vi "Populate gRPC Events.vi"(7 "RPC Method Parameters":T1[](array[typedef]), 8 "error in (no error)":errorcluster, 11 "Server class in":refnum<vi>) -> (0 "error out":errorcluster, 3 "Server class out":refnum<vi>)   [LabVIEW 2019, in "gRPC Template Creation Utility.lvlib"]
uses:
  gRPC Template Creation Utility.lvlib
  TypeDefs/RPC Method Parameters.ctl
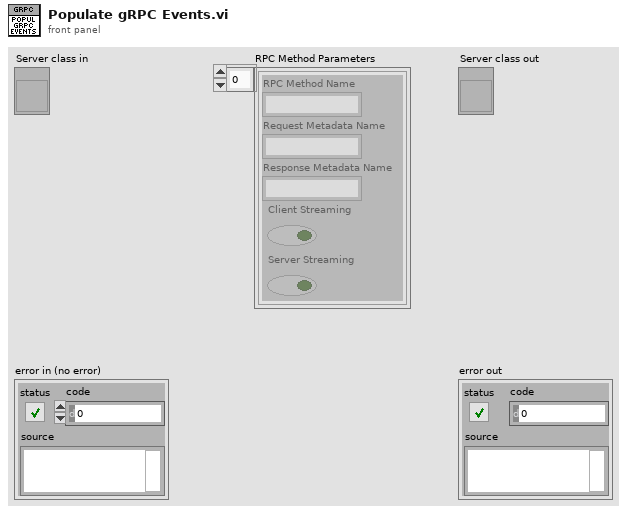
[diagram p1: front panel]
types:
  T1 = typedef "gRPC Template Creation Utility.lvlib/RPC Method Parameters.ctl" = cluster{"RPC Method Name":string, "Request Metadata Name":string, "Response Metadata Name":string, "Client Streaming":bool, "Server Streaming":bool}
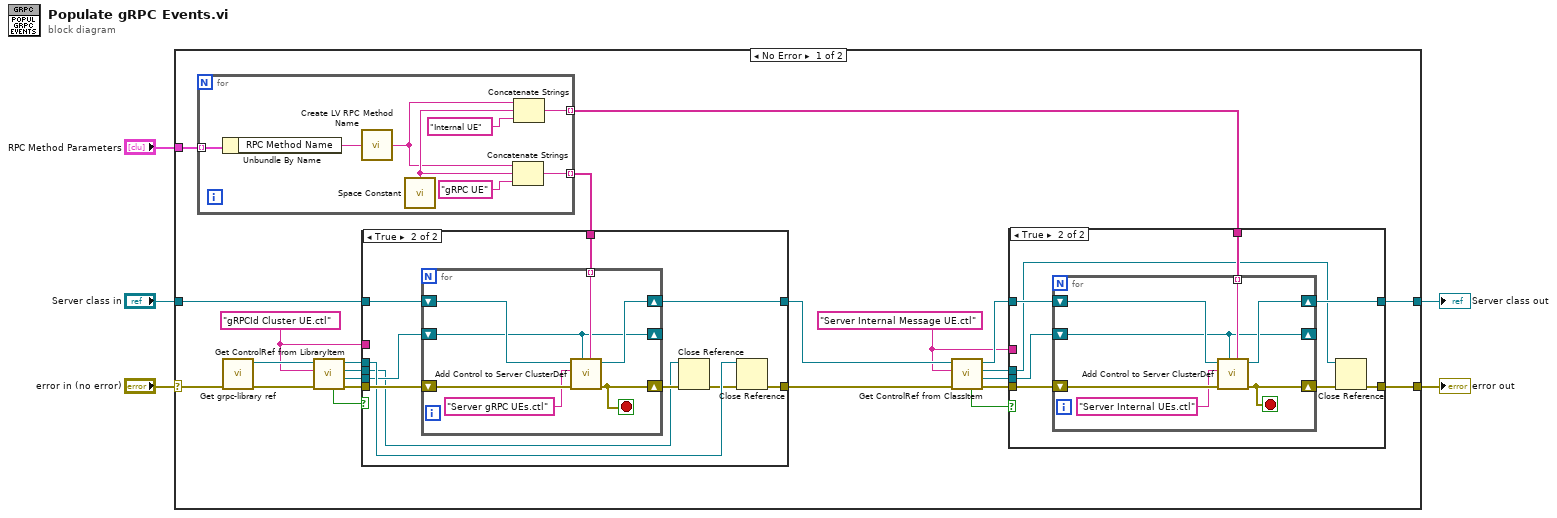
[diagram p0: block diagram]
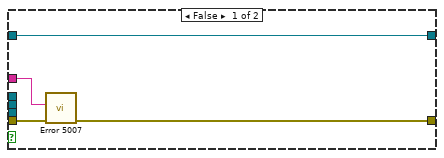
[diagram p2: hidden frame]
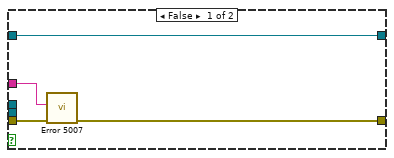
[diagram p3: hidden frame]
diagram:
  n1 = case shown="No Error" "error in (no error)" {
    selector: "error in (no error)" -> [w19 w77]
    tunnel: [w15 w77] -> w5
    tunnel: [w28 w78] -> w4
    tunnel: "Server class in" -> [w12 w78]
    tunnel: "RPC Method Parameters" -> [w18 _]
    frame No Error {
      w14 = "Server Internal Message UE.ctl" ("Item Name")
      w13 = "gRPCId Cluster UE.ctl" ("y")
      n2 = for {
        tunnel: w18 -> [w76] mode=indexing
        tunnel: [w74] -> w17 mode=indexing
        tunnel: [w72] -> w16 mode=indexing
        n3 = Unbundle By Name(w76) -> ("RPC Method Name"=w70:string)
        n4 = call "Create LV RPC Method Name.vi"("Proto Parser RPC Method Name in"=w70) -> ("LV RPC Method Name out"=w69:string)
        n5 = call <vilib>:"Space Constant.vi"() -> ("String"=w71:string)
        n6 = Concatenate Strings(w69, w71, "gRPC UE" ("string")) -> (w74:string)
        n7 = Concatenate Strings(w69, w71, "Internal UE" ("string")) -> (w72:string)
      }
      n8 = call "Get grpc-library ref.vi"("error in"=w19) -> ("error out"=w21:errorcluster, "Library out"=w20:refnum<vi>)  [unwired: 9 in]
      n9 = call "Get ControlRef from LibraryItem.vi"("error in (no error)"=w21, "Control Name"=w13, "Library item in"=w20) -> ("error out"=w26:errorcluster, "Control ref out"=w7:refnum<vi>, "VI ref out"=w6:refnum<vi>, "Library item out"=w25:refnum<vi>, "Found?"=w8:bool)  [unwired: 4 in]
      n10 = case shown="True" w8 {
        tunnel: [w29 w42] -> w27
        tunnel: w12 -> [w32 w41]
        tunnel: w26 -> [w31 w40]
        tunnel: w25 -> [_ w39]
        tunnel: w7 -> [_ w37]
        tunnel: [w32 w35] -> w22
        tunnel: w17 -> [_ w34]
        tunnel: w13 -> [w30 _]
        tunnel: w6 -> [_ w33]
        frame False {
          n11 = call "Error 5007.vi"("error in (no error)"=w31, "Target ClusterDef Name"=w30) -> ("error out"=w29:errorcluster)  [unwired: 9 in]
        }
        frame True {
          n12 = for {
            shift-right: [w45] -> w36
            shift-left: w40 -> [w49]
            tunnel: w34 -> [w47] mode=indexing
            shift-right: [w46] -> w35
            shift-left: w41 -> [w48]
            shift-right: [w43] -> _
            shift-left: w37 -> [w43]
            stop <- w45 stop-if-true
            n13 = call "Add Control to Server ClusterDef.vi"("New Control Label"=w47, "Source Control ref in"=w43, "error in (no error)"=w49, "Target ClusterDef Name"="Server gRPC UEs.ctl" ("Item Name"), "Server class in"=w48) -> ("error out"=w45:errorcluster, "Server class out"=w46:refnum<vi>)  [unwired: 5 in]
          }
          n14 = Close Reference(reference=w33, error in (no error)=w36) -> (error out=w38:errorcluster)
          n15 = Close Reference(reference=w39, error in (no error)=w38) -> (error out=w42:errorcluster)
        }
      }
      n16 = call "Get ControlRef from ClassItem.vi"("error in (no error)"=w27, "item name"=w14, "class in"=w22) -> ("error out"=w24:errorcluster, "control"=w10:refnum<vi>, "VI ref out"=w9:refnum<vi>, "class out"=w23:refnum<vi>, "found"=w11:bool)  [unwired: 4 in]
      n17 = case shown="True" w11 {
        tunnel: [w53 w61] -> w28
        tunnel: w10 -> [_ w60]
        tunnel: w24 -> [w52 w59]
        tunnel: w23 -> [w53 w58]
        tunnel: w16 -> [_ w57]
        tunnel: [w51 w55] -> w15
        tunnel: w14 -> [w50 _]
        tunnel: w9 -> [_ w54]
        frame False {
          n18 = call "Error 5007.vi"("error in (no error)"=w52, "Target ClusterDef Name"=w50) -> ("error out"=w51:errorcluster)  [unwired: 9 in]
        }
        frame True {
          n19 = for {
            tunnel: w57 -> [w66] mode=indexing
            shift-right: [w65] -> w61
            shift-left: w58 -> [w67]
            shift-right: [w64] -> w56
            shift-left: w59 -> [w68]
            shift-right: [w63] -> _
            shift-left: w60 -> [w63]
            stop <- w64 stop-if-true
            n20 = call "Add Control to Server ClusterDef.vi"("New Control Label"=w66, "Source Control ref in"=w63, "error in (no error)"=w68, "Target ClusterDef Name"="Server Internal UEs.ctl", "Server class in"=w67) -> ("error out"=w64:errorcluster, "Server class out"=w65:refnum<vi>)  [unwired: 5 in]
          }
          n21 = Close Reference(reference=w54, error in (no error)=w56) -> (error out=w55:errorcluster)
        }
      }
    }
    frame Error {
    }
  }
  "error out" <- w5
  "Server class out" <- w4
